vi "Read Data From VS Engine.vi"(8 "error in":errorcluster, 10 "Read from VS Engine FIFO":refnum<k33>, 11 "Channel Pairs":T3 {"Block Data Refs"."Data Reference" format="%.0x"}) -> (0 "error out":errorcluster, 2 "Write Occured":bool, 3 "Channel Pairs":T3 {"Block Data Refs"."Data Reference" format="%.0x"})   [LabVIEW 2015, in "J1939 Addon Engine.lvlib" / "Inline Async API.lvlib"]
uses:
  Inline Async API.lvlib
  <vilib>/NI Veristand/Custom Device API/Block Data Reference.ctl
  <vilib>/NI Veristand/Custom Device API/Data Reference.ctl
  <vilib>/NI Veristand/Custom Device API/Global Data Refs.vi
  <vilib>/NI Veristand/Custom Device API/Custom Device API.lvlib
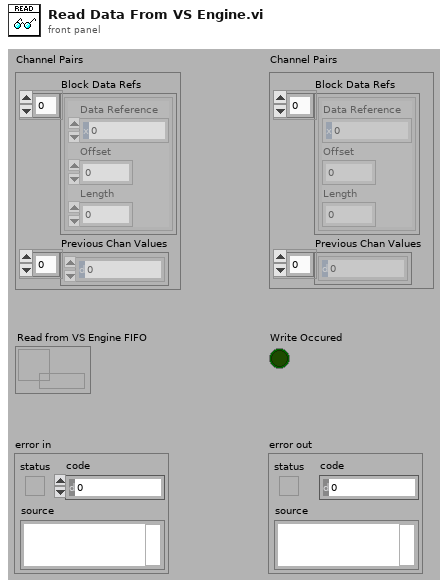
[diagram p1: front panel]
types:
  T1 = typedef "Custom Device API.lvlib/Block Data Reference.ctl" = cluster{"Data Reference":T2, "Offset":u64, "Length":u64}
  T2 = typedef "Custom Device API.lvlib/Data Reference.ctl" = i32
  T3 = cluster{"Block Data Refs":T1[], "Previous Chan Values":dbl[]}
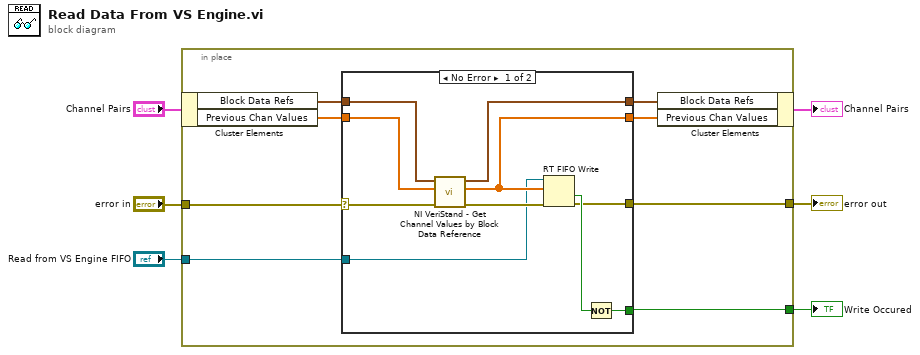
[diagram p0: block diagram]
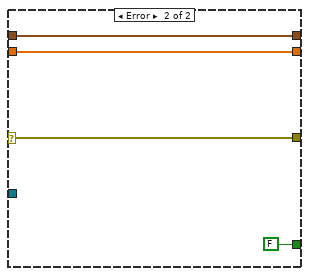
[diagram p2: hidden frame]
diagram:
  n1 = in-place {
    in-place-border: [w14] -> w6
    in-place-border: [w13] -> w5
    in-place-border: "error in" -> [w10]
    in-place-border: "Read from VS Engine FIFO" -> [w7]
    n2 = in-place-cluster #1("Channel Pairs") -> ("Block Data Refs"=w12:T1[], "Previous Chan Values"=w9:dbl[])
    n3 = case shown="No Error" w10 {
      selector: w10 -> [w21 w28]
      tunnel: [w22 w28] -> w14
      tunnel: [w16 w25] -> w8
      tunnel: [w23 FALSE ("C Read Occured?")] -> w13
      tunnel: w12 -> [w19 w26]
      tunnel: [w18 w26] -> w11
      tunnel: w9 -> [w17 w25]
      tunnel: w7 -> [w15 _]
      frame No Error {
        n4 = call <vilib>:"NI VeriStand - Get Channel Values by Block Data Reference.vi"("error in (no error)"=w21, "Values Array in"=w17, "Block Data Ref"=w19) -> ("error out"=w20:errorcluster, "Values Array out"=w16:dbl[], "Block Data Ref dup"=w18:T1[])  [unwired: 6 in]
        n5 = RT FIFO Write(0:w15, 1:w16, 3:w20) -> (10:w24:bool, 11:w22:errorcluster)  [unwired: 2 in, 2 out]
        n6 = Not(x=w24) -> (.not. x?=w23:bool)
      }
      frame Error {
      }
    }
    n7 = in-place-cluster #1("Block Data Refs"=w11, "Previous Chan Values"=w8) -> (→"Channel Pairs":T3)
  }
  "error out" <- w6
  "Write Occured" <- w5
